vi "Read Property.vi"(8 "error in (no error)":errorcluster, 11 "Node Ptr":T1 format="%.0x") -> (0 "error out":errorcluster, 3 "Node Ptr out":T1 format="%.0x")   [LabVIEW 2016, in "UDP-Custom-Device System Explorer.lvlib"]
uses:
  UDP-Custom-Device System Explorer.lvlib
  <vilib>/NI Veristand/Custom Device API/Custom Device Item Ref.ctl
  <vilib>/NI VeriStand/Custom Device API/Custom Device API.lvlib
  <vilib>/NI Veristand/Custom Device API/Get Item Property (Boolean).vi
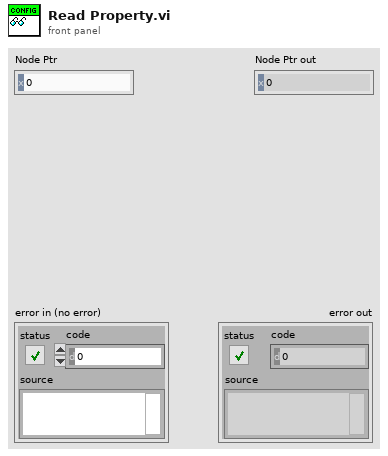
[diagram p1: front panel]
types:
  T1 = typedef "Custom Device API.lvlib/Custom Device Item Ref.ctl" = u64
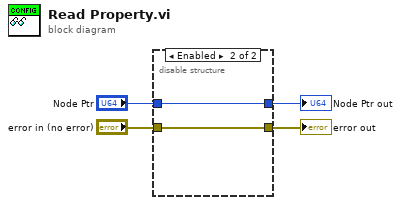
[diagram p0: block diagram]
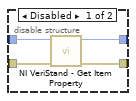
[diagram p2: hidden frame]
diagram:
  n1 = disable-structure shown="Enabled" {
    disable-tunnel: "error in (no error)" -> [w8 w9]
    disable-tunnel: "Node Ptr" -> [w7 w10]
    disable-tunnel: [w6 w10] -> w2
    disable-tunnel: [w5 w9] -> w1
    frame Disabled {
      n2 = call-poly <vilib>:"NI VeriStand - Get Item Property.vi"("error in (no error)"=w8, "Item Ref in"=w7) -> ("error out"=w5:errorcluster, "Item Ref out"=w6:T1)  [unwired: 6 in, 2 out]
    }
    frame Enabled {
    }
  }
  "error out" <- w1
  "Node Ptr out" <- w2
